vi "readASIC_param.vi"() -> ()   [LabVIEW 2009]
panel:
  out "Numeric 2":i32
  out "Numeric":i32
  out "Array":i32[][](array[numeric])
  out "size(s) 2":i32[](array[numeric])
  out "Array 3":dbl[](array[numeric])
  out "size(s)":i32
  out "index of element":i32
  out "array":dbl[][](array[numeric])
  out "error out":errorcluster
  in  "count":i32
  in  "error in":errorcluster
  in  "file (use dialog)":path
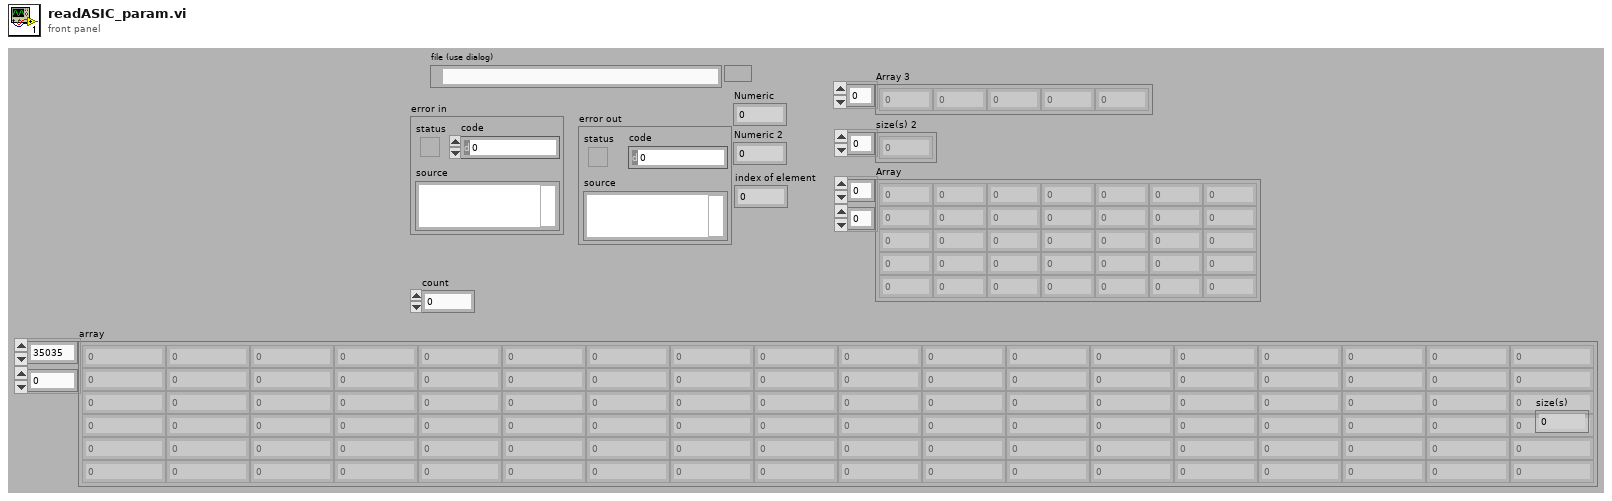
[diagram p1: front panel]
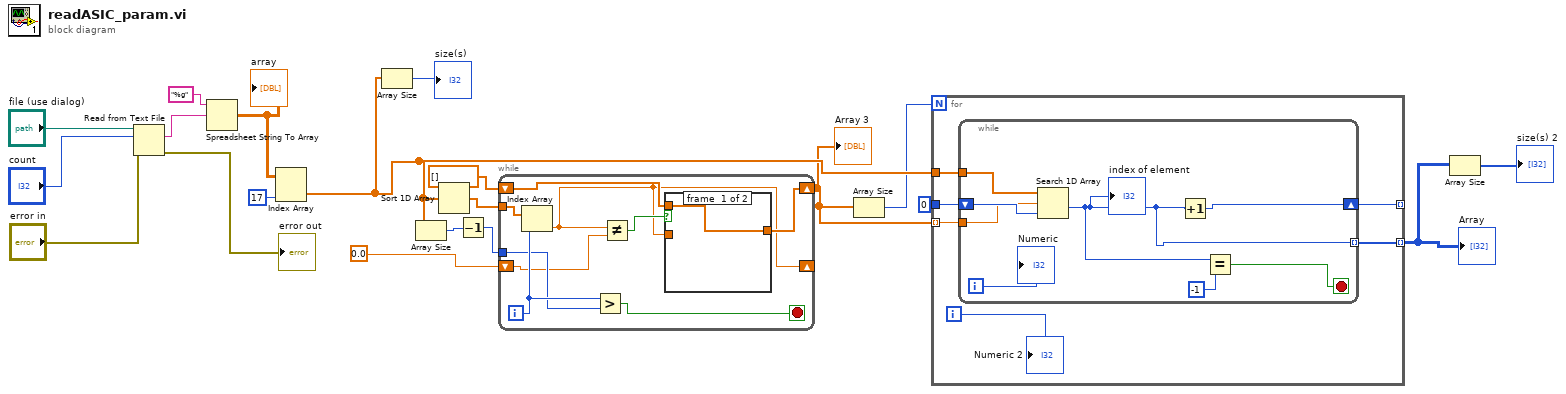
[diagram p0: block diagram]
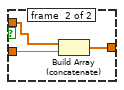
[diagram p2: hidden frame]
diagram:
  n1 = Read from Text File(file (use dialog)="file (use dialog)", count="count", error in="error in") -> (text=w16:string, error out=→"error out":errorcluster)  [unwired: 1 in, 2 out]
  n2 = Spreadsheet String To Array(format string="%g", spreadsheet string=w16) -> (array=w14:dbl[][])  [unwired: 2 in]
  "array" <- w14
  n3 = Index Array(array=w14, index (col)=17 ("disabled index (col)")) -> (element=w12:dbl[])  [unwired: 1 in]
  n4 = Array Size(array=w12) -> (size(s)=→"size(s)":i32)
  n5 = Array Size(array=w12) -> (size(s)=w8:i32)
  n6 = Sort 1D Array(array=w12) -> (sorted array=w5:dbl[])
  n7 = Decrement(x=w8) -> (x-1=w7:i32)
  n8 = while {
    tunnel: w5 -> [w29]
    shift-right: [w21] -> _
    shift-left: 0.0 ("element") -> [w25]
    tunnel: w7 -> [w27]
    shift-right: [w22] -> w3
    shift-left: dbl[] [] -> [w23]
    i -> [w28]
    stop <- w26 stop-if-true
    n9 = Index Array(array=w29, index=w28) -> (element=w21:dbl)
    n10 = Greater?(x=w28, y=w27) -> (0:w26:bool)
    n11 = Not Equal?(x=w21, y=w25) -> (x != y?=w24:bool)
    n12 = case shown="True" w24 {
      tunnel: w23 -> [w30 w33]
      tunnel: [w30 w32] -> w22
      tunnel: w21 -> [_ w31]
      frame #0 {
      }
      frame #1 {
        n13 = Build Array (concatenate)(w33, w31) -> (w32:dbl[])
      }
    }
  }
  "Array 3" <- w3
  n14 = Array Size(array=w3) -> (size(s)=w4:i32)
  n15 = for {
    N: w4 -> [_]
    tunnel: w12 -> [w37]
    tunnel: [w36] -> w2 mode=indexing
    tunnel: w3 -> [w35] mode=indexing
    tunnel: 0 ("index of element") -> [w39]
    tunnel: [w38] -> _ mode=indexing
    i -> [w34]
    n16 = while {
      tunnel: w37 -> [w45]
      tunnel: [w43] -> w36 mode=indexing
      tunnel: w35 -> [w44]
      shift-right: [w46] -> w38
      shift-left: w39 -> [w47]
      i -> [w40]
      stop <- w41 stop-if-true
      n17 = Search 1D Array(1D array=w45, element=w44, start index (0)=w47) -> (index of element=w43:i32)
      "index of element" <- w43
      n18 = Increment(x=w43) -> (x+1=w46:i32)
      n19 = Equal?(x=w43, y=-1) -> (x = y?=w41:bool)
      "Numeric" <- w40
    }
    "Numeric 2" <- w34
  }
  "Array" <- w2
  n20 = Array Size(array=w2) -> (size(s)=→"size(s) 2":i32[])
